vi "GetTeleopQueue.vi"(8 "error in (no error)":errorcluster) -> (0 "error out":errorcluster, 3 "notifier out":refnum<notifier>)   [LabVIEW 2013]
uses:
  TeleopInstruction.ctl
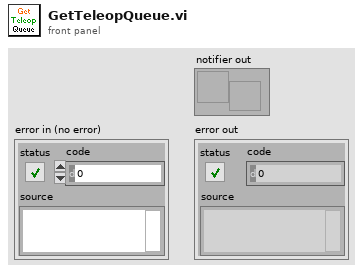
[diagram p1: front panel]
types:
  T1 = typedef "TeleopInstruction.ctl" = cluster{"cDriveLeft":dbl, "cDriveRight":dbl, "cHalfDrive":bool, "cStraightDrive":bool, "cSonicShifter":bool}
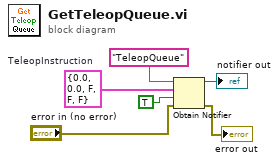
[diagram p0: block diagram]
diagram:
  w2 = T1 {"cDriveLeft"=0.0, "cDriveRight"=0.0, "cHalfDrive"=FALSE, "cStraightDrive"=FALSE, "cSonicShifter"=FALSE}  # TeleopInstruction
  n1 = Obtain Notifier(name (unnamed)="TeleopQueue", notification data type=w2, create if not found? (T)=TRUE, error in (no error)="error in (no error)") -> (notifier out=→"notifier out":refnum<notifier>, error out=→"error out":errorcluster)  [unwired: 1 out]
